vi "GOOP_AddingClassTemplateDialog.vi"(9 "ShortName(Could be used in for INI Sections)":string="Native", 10 "TranslatedProviderName":string="By Value", 11 "FolderPathOut":path=path "C:/Program Files (x86)/National Instruments/LabVIEW 2020/resource/Framework/Providers/Open_GDS/ClassProviders/Provider_LvNativeClass/Templates") -> (3 "Cancelled":bool)   [LabVIEW 2020]
panel:
  out "Method1 2":string
  out "Text 3":string
  out "Method2":string
  out "Method1":string
  in  "Custom Templates":path[](array[path])
  in  "Cancel":bool
  in  "Save":bool
  out "Text":string
  out "Text 2":string
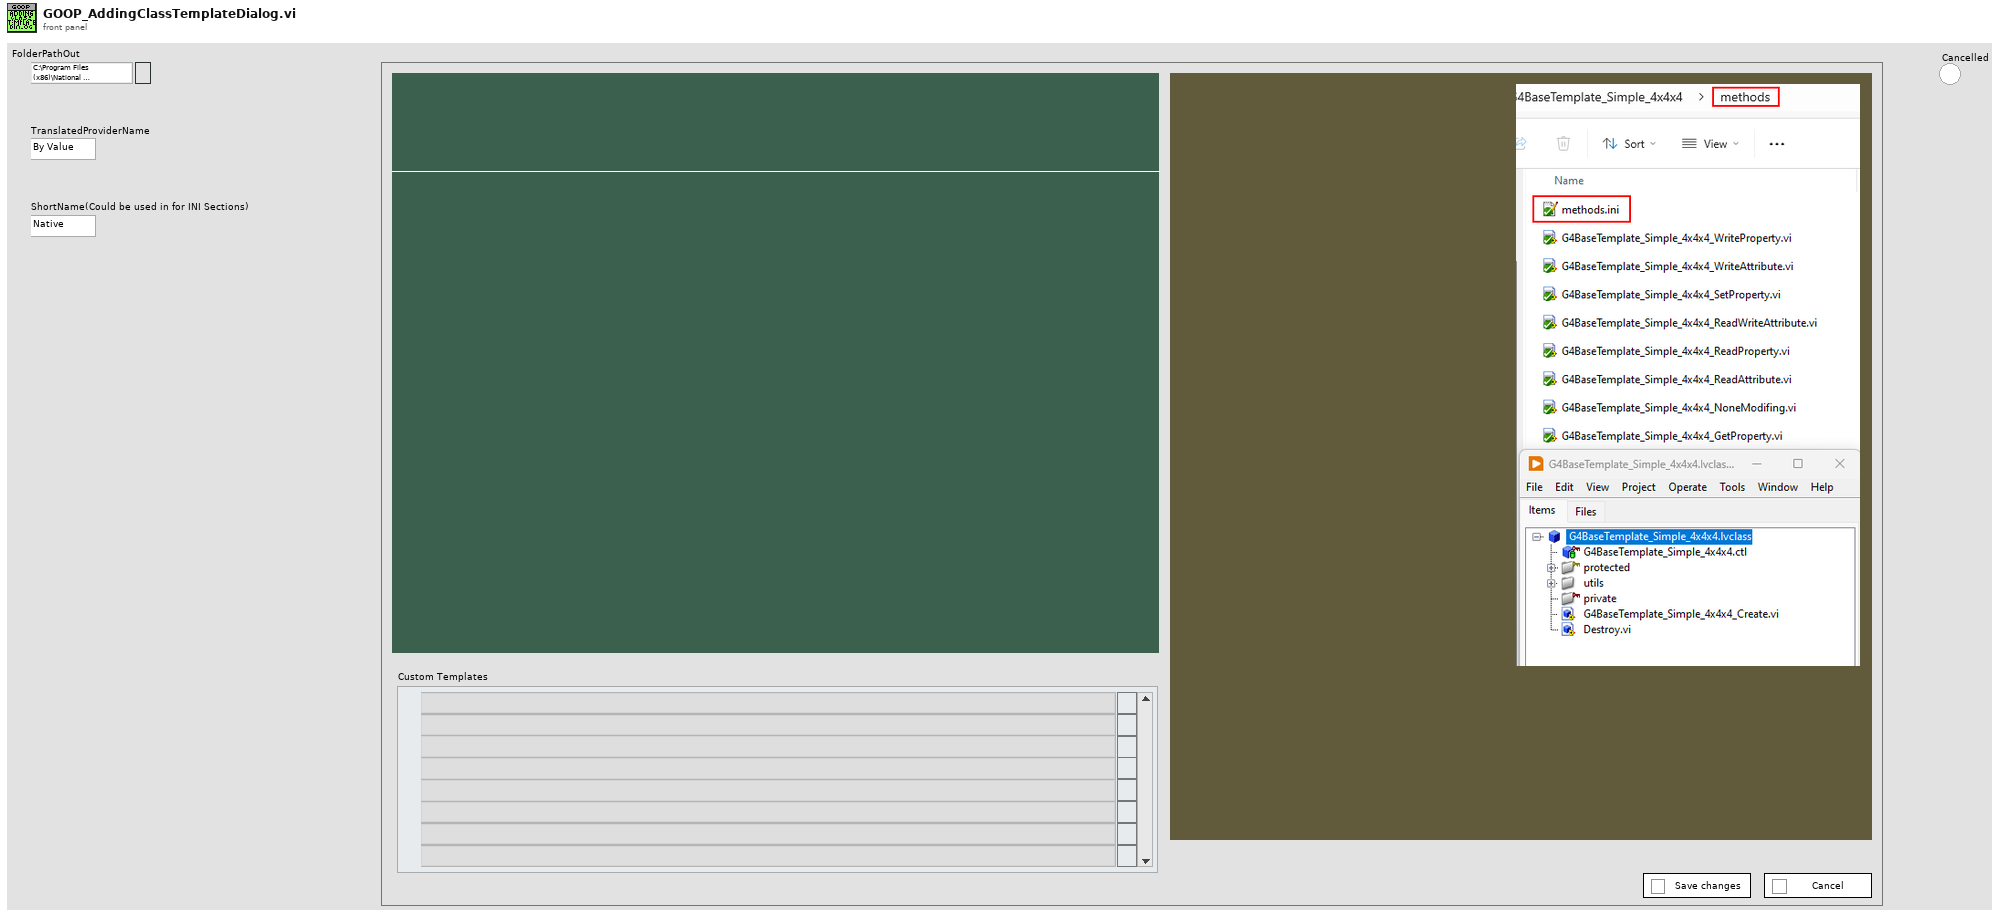
[diagram p1: front panel]
types:
  T1 = enum8{"Enabled", "Disabled", "Disabled and Grayed Out"}
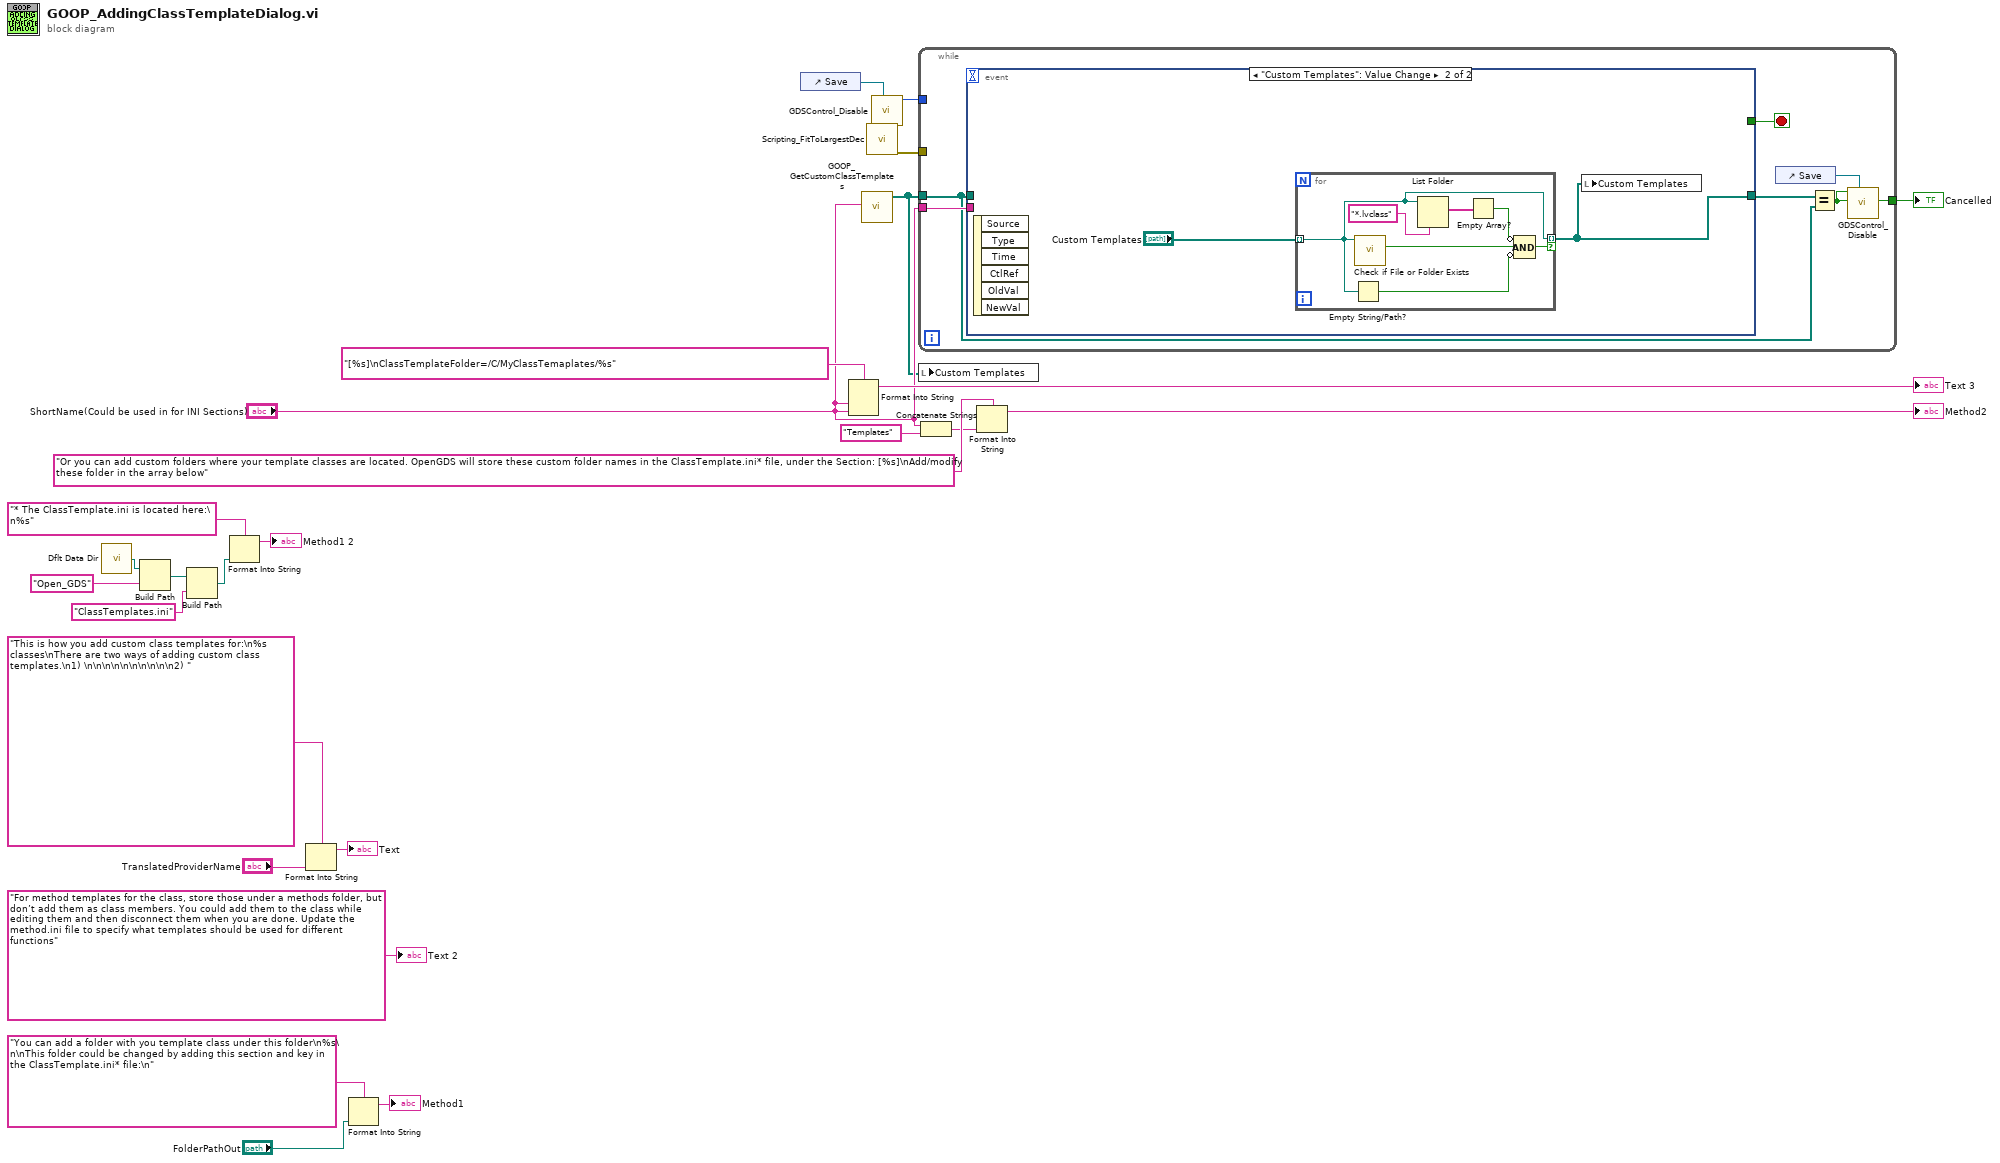
[diagram p0: block diagram]
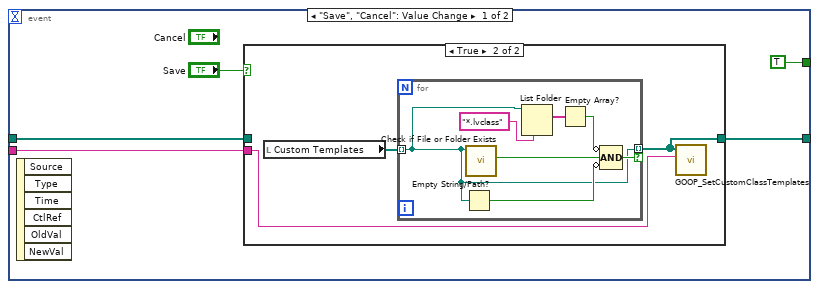
[diagram p2: hidden frame]
diagram:
  n1 = call <vilib>:"Dflt Data Dir.vi"() -> ("App:Default Data Directory"=w24:path)
  n2 = Build Path(base path=w24, name or relative path="Open_GDS") -> (appended path=w22:path)
  n3 = Build Path(base path=w22, name or relative path="ClassTemplates.ini") -> (appended path=w7:path)
  n4 = Format Into String(format string="* The ClassTemplate.ini is located here:\n%s", w7) -> (resulting string=→"Method1 2":string)  [unwired: 2 in, 1 out]
  n5 = Format Into String(format string="This is how you add custom class templates for:\n%s classes\nThere are two ways of adding custom class templates.\n1) \n\n\n\n\n\n\n\n\n\n2) ", "TranslatedProviderName") -> (resulting string=→"Text":string)  [unwired: 2 in, 1 out]
  n6 = Format Into String(format string="You can add a folder with you template class under this folder\n%s\n\nThis folder could be changed by adding this section and key in the ClassTemplate.ini* file:\n", "FolderPathOut") -> (resulting string=→"Method1":string)  [unwired: 2 in, 1 out]
  n7 = control-ref of="Save"() -> (w3:refnum<vi>)
  n8 = Format Into String(format string="[%s]\nClassTemplateFolder=/C/MyClassTemaplates/%s" ("Text 3"), "ShortName(Could be used in for INI Sections)", "ShortName(Could be used in for INI Sections)") -> (resulting string=→"Text 3":string)  [unwired: 2 in, 1 out]
  n9 = call <resource>:"GOOP_GetCustomClassTemplates.vi"("ClassType"="ShortName(Could be used in for INI Sections)") -> ("CustomTemplates"=w4:path[])  [unwired: 10 in]
  n10 = call <resource>:"Scripting_FitToLargestDec.vi"() -> ("error out"=w1:errorcluster)  [unwired: 6 in, 1 out]
  n11 = call <resource>:"GDSControl_Disable.vi"("ControlRefnum(IgnoreIfNotWired)"=w3) -> ("Enable Property"=w2:T1)  [unwired: 10 in]
  n12 = while {
    tunnel: "ShortName(Could be used in for INI Sections)" -> [w32]
    tunnel: [w28] -> w5
    tunnel: w4 -> [w30]
    tunnel: w2 -> [_]
    tunnel: w1 -> [_]
    stop <- w29 stop-if-true
    n13 = event shown="[1] \"Custom Templates\": Value Change" {
      selector: _ -> [_ _]
      dyn-events: _ -> [_ _]
      timeout: _ -> [_ _]
      tunnel: w32 -> [w37 _]
      tunnel: [w35 w49] -> w31
      tunnel: w30 -> [w34 _]
      tunnel: [TRUE _] -> w29
      event "Save", "Cancel": Value Change {
        n14 = event-data() -> ()  [unwired: 1 in, 6 out]
        n15 = case shown="True" "Save" {
          tunnel: w37 -> [_ w41]
          tunnel: [w38 w40] -> w35
          tunnel: w34 -> [w38 _]
          frame False {
          }
          frame True {
            n16 = local read "Custom Templates"() -> (w39:path[])
            n17 = for {
              tunnel: w39 -> [w45] mode=indexing
              tunnel: [w45] -> w40 mode=indexing if=w46
              n18 = Empty String/Path?(string/path=w45) -> (empty?=w47:bool)
              n19 = call <vilib>:"Check if File or Folder Exists.vi"("path"=w45) -> ("file or folder exists?"=w48:bool)  [unwired: 8 in, 2 out]
              n20 = List Folder(path=w45, pattern="*.lvclass") -> (filenames=w43:string[])  [unwired: 2 in, 3 out]
              n21 = Empty Array?(array=w43) -> (empty?=w42:bool)
              n22 = Compound Arithmetic op=AND(invert w42, w48, invert w47) -> (w46:bool)
            }
            n23 = call <resource>:"GOOP_SetCustomClassTemplates.vi"("ClassType"=w41, "CustomTemplates"=w40) -> ()  [unwired: 10 in]
          }
        }
      }
      event "Custom Templates": Value Change {
        n24 = event-data() -> ()  [unwired: 1 in, 6 out]
        n25 = for {
          tunnel: "Custom Templates" -> [w54] mode=indexing
          tunnel: [w54] -> w49 mode=indexing if=w55
          n26 = Empty String/Path?(string/path=w54) -> (empty?=w56:bool)
          n27 = call <vilib>:"Check if File or Folder Exists.vi"("path"=w54) -> ("file or folder exists?"=w57:bool)  [unwired: 8 in, 2 out]
          n28 = List Folder(path=w54, pattern="*.lvclass") -> (filenames=w52:string[])  [unwired: 2 in, 3 out]
          n29 = Empty Array?(array=w52) -> (empty?=w51:bool)
          n30 = Compound Arithmetic op=AND(invert w51, w57, invert w56) -> (w55:bool)
        }
        n31 = local write "Custom Templates"(w49) -> ()
      }
    }
    n32 = control-ref of="Save"() -> (w27:refnum<vi>)
    n33 = Equal?(x=w31, y=w30) -> (x = y?=w28:bool)
    n34 = call <resource>:"GDSControl_Disable.vi"("ControlRefnum(IgnoreIfNotWired)"=w27, "Disasble(True)"=w28) -> ()  [unwired: 9 in, 1 out]
  }
  "Cancelled" <- w5
  n35 = local write "Custom Templates"(w4) -> ()
  n36 = Concatenate Strings("ShortName(Could be used in for INI Sections)", "Templates" ("string")) -> (w17:string)
  n37 = Format Into String(format string="Or you can add custom folders where your template classes are located. OpenGDS will store these custom folder names in the ClassTemplate.ini* file, under the Section: [%s]\nAdd/modify these folder in the array below", w17) -> (resulting string=→"Method2":string)  [unwired: 2 in, 1 out]
  "Text 2" <- "For method templates for the class, store those under a methods folder, but don’t add them as class members. You could add them to the class while editing them and then disconnect them when you are done. Update the method.ini file to specify what templates should be used for different functions" ("Text 2")
